vi "Get Font.vi"(0 "Font":refnum<class "Font Class.lvclass">, 7 "Font IN":T1={"Name"="Helvetica", "Size"=12.0, "Color"=0, "Style"={"Bold"=FALSE, "Italic"=FALSE, "Underline"=FALSE, "Strikeout"=FALSE}, "Type"={"Type&direction"=enum."Select", "Embedded"=FALSE, "Encoding"=""}}, 11 "error in (no error)":errorcluster) -> (4 "Font duplicate":refnum<class "Font Class.lvclass">, 6 "Font":refnum<k24>, 8 "Font OUT":T1={"Name"="Helvetica", "Size"=12.0, "Color"=0, "Style"={"Bold"=FALSE, "Italic"=FALSE, "Underline"=FALSE, "Strikeout"=FALSE}, "Type"={"Type&direction"=enum."Select", "Embedded"=FALSE, "Encoding"=""}}, 10 "Font Size":T2=12.0, 15 "error out":errorcluster)   [LabVIEW 2019, in "Exaprom PDF.lvlib" / "Font Class.lvclass"]
doc: "Version 1.0\nDeveloped by Jean-Marc Simard\nCopyright © 2012, Exaprom Inc.\nAll rights reserved.\nLicense: BSD\n\nWith iTextSharp 4.1.6 (http://itextsharp.sourceforge.net)\nunder Mozilla Public License Version 1.1\n(http://www.mozilla.org/MPL/MPL-1.1.html)"
uses:
  Font Class.lvclass
  Controls/Font Controls/Font complete cluster.ctl
  Controls/Font Controls/Font size.ctl
  Controls/Font Controls/Font color.ctl
  Controls/Font Controls/Type and encoding.ctl
  Controls/Text Controls/Unicode/Type and run direction.ctl
  C:/work/niobrara_lv/labview pdf writer fixing/DLL/itextsharp.dll
  DLL/itextsharp.dll
  Exaprom PDF.lvlib
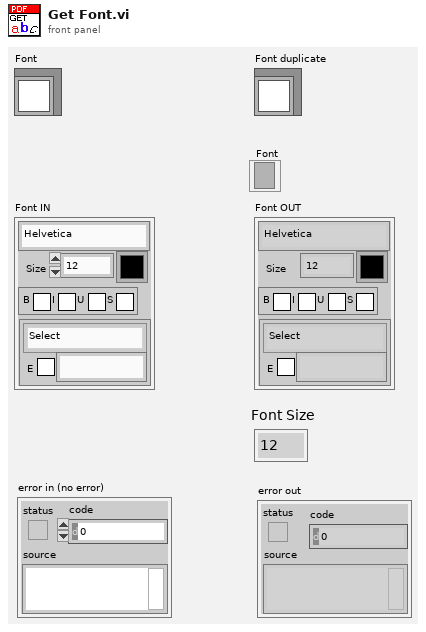
[diagram p1: front panel]
types:
  T1 = typedef "Exaprom PDF.lvlib/Font complete cluster.ctl" = cluster{"Name":string, "Size":T2, "Color":T3, "Style":cluster{"Bold":bool, "Italic":bool, "Underline":bool, "Strikeout":bool}, "Type":T4}
  T2 = typedef "Exaprom PDF.lvlib/Font size.ctl" = sgl
  T3 = typedef "Exaprom PDF.lvlib/Font color.ctl" = u32
  T4 = typedef "Exaprom PDF.lvlib/Type and encoding.ctl" = cluster{"Type&direction":T5, "Embedded":bool, "Encoding":string}
  T5 = typedef "Exaprom PDF.lvlib/Type and run direction.ctl" = enum16{"Select", "ASCII", "UTF-16", "UTF-16 (default)", "UTF-16 (LTR)", "UTF-16 (RTL)"}
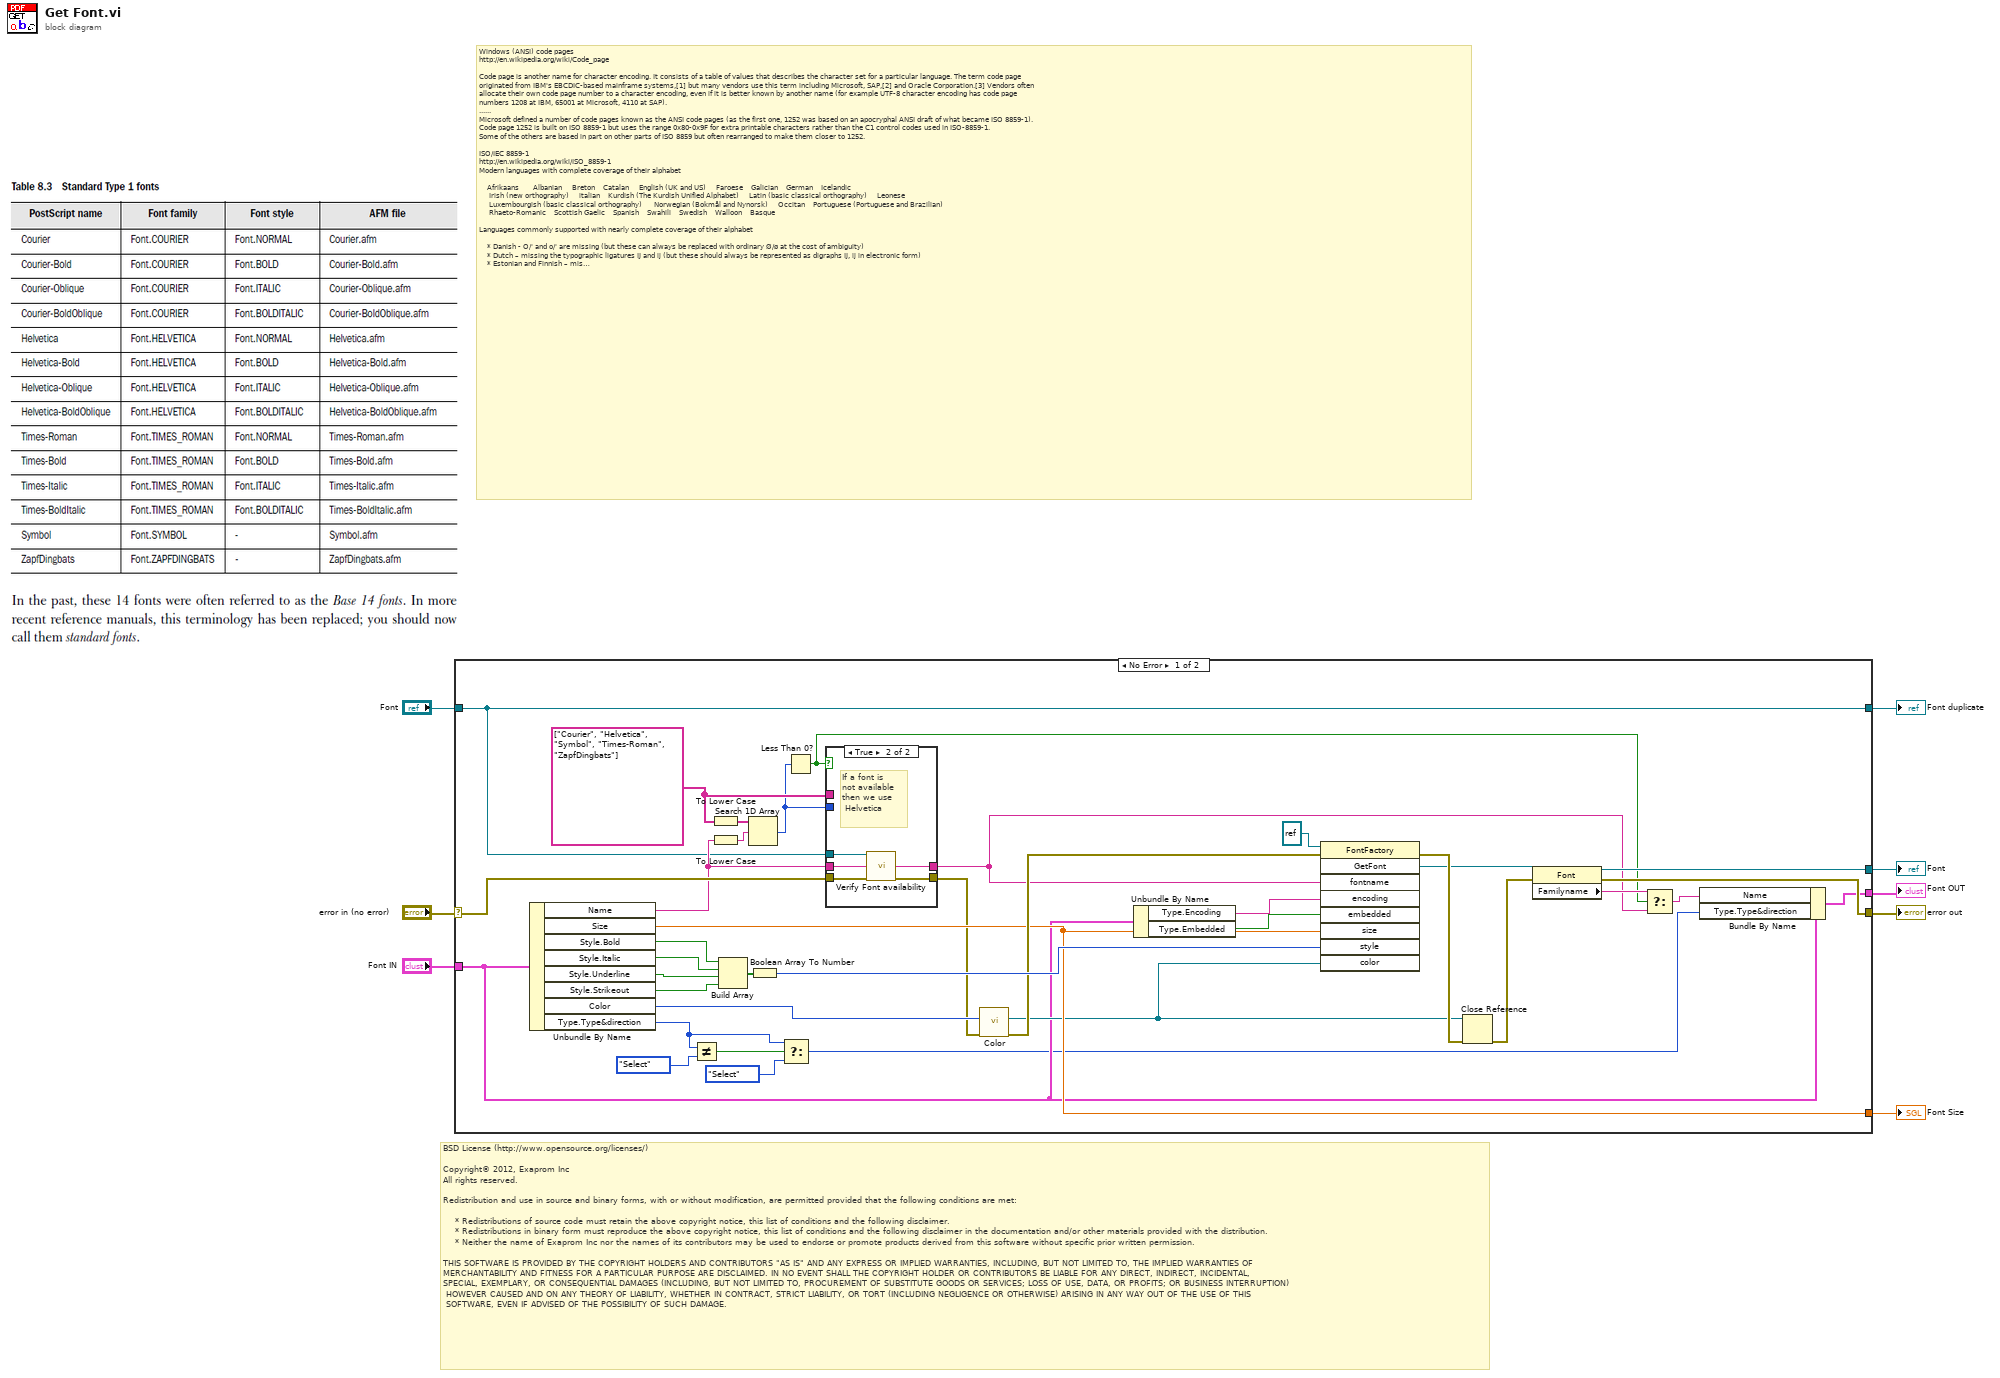
[diagram p0: block diagram]
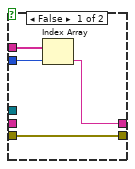
[diagram p2: hidden frame]
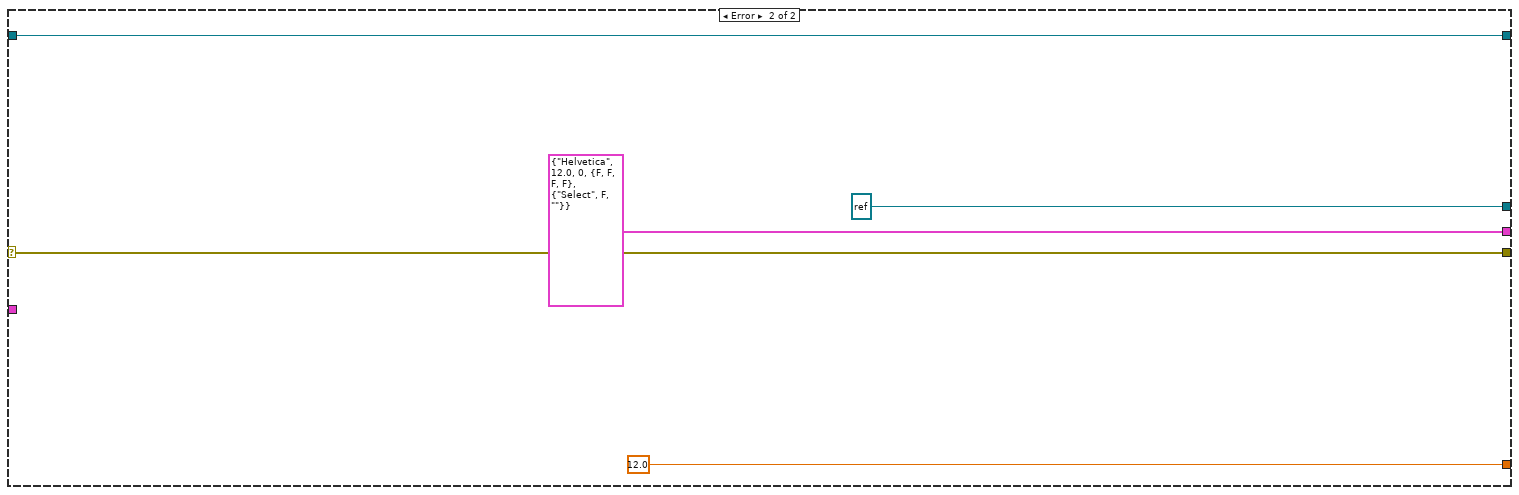
[diagram p3: hidden frame]
diagram:
  # "Windows (ANSI) code pages\nhttp://en.wikipedia.org/wiki/Code_page\n\nCode page is another name for character encoding. It consists of a table of values that describes the character set for a particular language. The term code page\noriginated from IBM's EBCDIC-based mainframe systems,[1] but many vendors use this term including Microsoft, SAP,[2] and Oracle Corporation.[3] Vendors often\nallocate their own code page number to a character encoding, even if it is better known by another name (for example UTF-8 character encoding has code page \nnumbers 1208 at IBM, 65001 at Microsoft, 4110 at SAP).\n......\nMicrosoft defined a number of code pages known as the ANSI code pages (as the first one, 1252 was based on an apocryphal ANSI draft of what became ISO 8859-1). \nCode page 1252 is built on ISO 8859-1 but uses the range 0x80-0x9F for extra printable characters rather than the C1 control codes used in ISO-8859-1. \nSome of the others are based in part on other parts of ISO 8859 but often rearranged to make them closer to 1252.\n\nISO/IEC 8859-1\nhttp://en.wikipedia.org/wiki/ISO_8859-1\nModern languages with complete coverage of their alphabet\n\n    Afrikaans       Albanian     Breton    Catalan     English (UK and US)     Faroese    Galician    German    Icelandic\n     Irish (new orthography)     italian    Kurdish (The Kurdish Unified Alphabet)     Latin (basic classical orthography)     Leonese\n     Luxembourgish (basic classical orthography)      Norwegian (Bokmål and Nynorsk)     Occitan    Portuguese (Portuguese and Brazilian)\n     Rhaeto-Romanic    Scottish Gaelic    Spanish    Swahili    Swedish    Walloon    Basque\n\nLanguages commonly supported with nearly complete coverage of their alphabet\n\n    * Danish - O/' and o/' are missing (but these can always be replaced with ordinary Ø/ø at the cost of ambiguity)\n    * Dutch – missing the typographic ligatures IJ and ij (but these should always be represented as digraphs IJ, ij in electronic form)\n    * Estonian and Finnish – missing Š, š, Ž, ž, which can only occur in loanwords (the missing characters are often replaced by digraphs Sh, sh, Zh, zh) (Windows-1252 and ISO-8859-15 do contain these)\n    * French – missing the ligatures Œ and œ as well as the very rare Ÿ (they are generally replaced by digraphs OE and oe, and Y without the diaeresis) (Windows-1252 and ISO-8859-15 do contain these)\n    * Hungarian – missing O\", o\", U\", u\"\n    * Latin (classical language written using macrons) – missing A-, a-, E-, e-, I-, i-, O-, o-, U-, u-\n    * Welsh – missing W^, w^, Y^, y^ (ISO-8859-14 does contain these)\n    * Maori – missing A-, a-, E-, e-, I-, i-, O-, o-, U-, u-"
  # "BSD License (http://www.opensource.org/licenses/)\n\nCopyright© 2012, Exaprom Inc\nAll rights reserved.\n\nRedistribution and use in source and binary forms, with or without modification, are permitted provided that the following conditions are met:\n\n    * Redistributions of source code must retain the above copyright notice, this list of conditions and the following disclaimer.\n    * Redistributions in binary form must reproduce the above copyright notice, this list of conditions and the following disclaimer in the documentation and/or other materials provided with the distribution.\n    * Neither the name of Exaprom Inc nor the names of its contributors may be used to endorse or promote products derived from this software without specific prior written permission.\n\nTHIS SOFTWARE IS PROVIDED BY THE COPYRIGHT HOLDERS AND CONTRIBUTORS \"AS IS\" AND ANY EXPRESS OR IMPLIED WARRANTIES, INCLUDING, BUT NOT LIMITED TO, THE IMPLIED WARRANTIES OF \nMERCHANTABILITY AND FITNESS FOR A PARTICULAR PURPOSE ARE DISCLAIMED. IN NO EVENT SHALL THE COPYRIGHT HOLDER OR CONTRIBUTORS BE LIABLE FOR ANY DIRECT, INDIRECT, INCIDENTAL,\nSPECIAL, EXEMPLARY, OR CONSEQUENTIAL DAMAGES (INCLUDING, BUT NOT LIMITED TO, PROCUREMENT OF SUBSTITUTE GOODS OR SERVICES; LOSS OF USE, DATA, OR PROFITS; OR BUSINESS INTERRUPTION)\n HOWEVER CAUSED AND ON ANY THEORY OF LIABILITY, WHETHER IN CONTRACT, STRICT LIABILITY, OR TORT (INCLUDING NEGLIGENCE OR OTHERWISE) ARISING IN ANY WAY OUT OF THE USE OF THIS\n SOFTWARE, EVEN IF ADVISED OF THE POSSIBILITY OF SUCH DAMAGE."
  n1 = case shown="No Error" "error in (no error)" {
    selector: "error in (no error)" -> [w28 w57]
    tunnel: [w31 refnum<k24> refnum ("GetFont")] -> w4
    tunnel: "Font IN" -> [w20 _]
    tunnel: [w32 T2 12.0 ("Size")] -> w6
    tunnel: [w45 w57] -> w5
    tunnel: [w30 T1 {"Name"="Helvetica", "Size"=12.0, "Color"=0, "Style"={"Bold"=FALSE, "Italic"=FALSE, "Underline"=FALSE, "Strikeout"=FALSE}, "Type"={"Type&direction"=enum."Select", "Embedded"=FALSE, "Encoding"=""}} ("Font OUT")] -> w3
    tunnel: "Font" -> [w14 w56]
    tunnel: [w14 w56] -> w1
    frame No Error {
      w24 = string[] ["Courier", "Helvetica", "Symbol", "Times-Roman", "ZapfDingbats"] ("Strings []")
      n2 = Unbundle By Name(w20) -> ("Name"=w25:string, "Size"=w32:T2, "Style.Bold"=w43:bool, "Style.Italic"=w42:bool, "Style.Underline"=w41:bool, "Style.Strikeout"=w40:bool, "Color"=w39:T3, "Type.Type&direction"=w11:T5)
      n3 = Not Equal?(x=w11, y=Type_and_run_direction."Select") -> (x != y?=w12:bool)
      n4 = To Lower Case(string=w24) -> (all lower case string=w34:string[])
      n5 = To Lower Case(string=w25) -> (all lower case string=w33:string)
      n6 = Build Array(w43, w42, w41, w40) -> (w44:bool[])
      n7 = Search 1D Array(1D array=w34, element=w33) -> (index of element=w23:i32)  [unwired: 1 in]
      n8 = Boolean Array To Number(Boolean array=w44) -> (number=w38:u32)
      n9 = Select(t=w11, s=w12, f=Type_and_run_direction."Select") -> (s? t:f=w9:T5)
      n10 = Less Than 0?(x=w23) -> (x < 0?=w15:bool)
      n11 = case shown="True" w15 {
        tunnel: [w46 w53] -> w16
        tunnel: w25 -> [_ w54]
        tunnel: w28 -> [w49 w52]
        tunnel: [w49 w51] -> w27
        tunnel: w24 -> [w48 _]
        tunnel: w23 -> [w47 _]
        tunnel: w14 -> [_ w50]
        frame False {
          n12 = Index Array(array=w48, index=w47) -> (element=w46:string)
        }
        frame True {
          # "If a font is \nnot available\nthen we use\n Helvetica"
          n13 = call "Verify Font availability.vi"("Font IN"=w50, "Font name"=w54, "error in (no error)"=w52) -> ("Font"=w53:string, "error out"=w51:errorcluster)  [unwired: 10 in, 1 out]
        }
      }
      n14 = call "Color.vi"("error in (no error)"=w27, "Color"=w39) -> ("error out"=w35:errorcluster, "Color"=w29:refnum<k24>)  [unwired: 8 out]
      n15 = Unbundle By Name(w20) -> ("Type.Encoding"=w21:string, "Type.Embedded"=w22:bool)
      n16 = invoke class="FontFactory" method="GetFont"(reference=refnum<k24> refnum, error in=w35, "fontname"=w16, "encoding"=w21, "embedded"=w22, "size"=w32, "style"=w38, "color"=w29) -> (error out=w36:errorcluster, "GetFont"=w19:refnum<k24>)  [unwired: 1 in, 7 out]
      n17 = Close Reference(reference=w29, error in (no error)=w36) -> (error out=w26:errorcluster)
      n18 = property class="Font"(reference=w19, error in=w26) -> (reference out=w31:refnum<k24>, error out=w45:errorcluster, "Familyname"=w18:string)
      n19 = Select(t=w18, s=w15, f=w16) -> (s? t:f=w17:string)
      n20 = Bundle By Name(cluster=w20, "Name"=w17, "Type.Type&direction"=w9) -> (w30:T1)
    }
    frame Error {
    }
  }
  "error out" <- w5
  "Font" <- w4
  "Font Size" <- w6
  "Font OUT" <- w3
  "Font duplicate" <- w1
